vi "Test Control Packets.vi"() -> (0 "error out":errorcluster)   [LabVIEW 2013]
uses:
  <vilib>/addons/_JKI Toolkits/Caraya/classes/Test/Test.lvclass
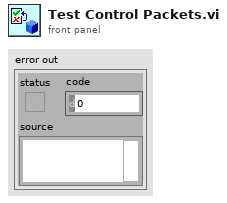
[diagram p1: front panel]
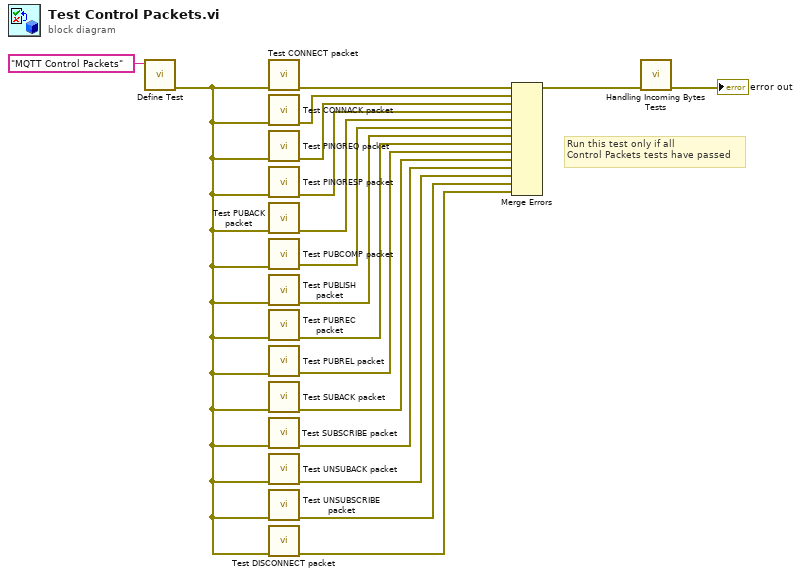
[diagram p0: block diagram]
diagram:
  # "Run this test only if all\nControl Packets tests have passed"
  n1 = call <vilib>:"Define Test.vi"("Label (VI Title)"="MQTT Control Packets") -> ("error out"=w1:errorcluster)  [unwired: 10 in]
  n2 = call "Test CONNECT packet.vi"("error in (no error)"=w1) -> ("error out"=w17:errorcluster)  [unwired: 10 in]
  n3 = call "Test CONNACK packet.vi"("error in (no error)"=w1) -> ("error out"=w16:errorcluster)  [unwired: 10 in]
  n4 = call "Test PINGREQ packet.vi"("error in (no error)"=w1) -> ("error out"=w15:errorcluster)  [unwired: 10 in]
  n5 = call "Test PINGRESP packet.vi"("error in (no error)"=w1) -> ("error out"=w14:errorcluster)  [unwired: 10 in]
  n6 = call "Test PUBACK packet.vi"("error in (no error)"=w1) -> ("error out"=w11:errorcluster)  [unwired: 10 in]
  n7 = call "Test PUBCOMP packet.vi"("error in (no error)"=w1) -> ("error out"=w10:errorcluster)  [unwired: 10 in]
  n8 = call "Test PUBLISH packet.vi"("error in (no error)"=w1) -> ("error out"=w9:errorcluster)  [unwired: 10 in]
  n9 = call "Test PUBREC packet.vi"("error in (no error)"=w1) -> ("error out"=w8:errorcluster)  [unwired: 10 in]
  n10 = call "Test PUBREL packet.vi"("error in (no error)"=w1) -> ("error out"=w7:errorcluster)  [unwired: 10 in]
  n11 = call "Test SUBACK packet.vi"("error in (no error)"=w1) -> ("error out"=w6:errorcluster)  [unwired: 10 in]
  n12 = call "Test SUBSCRIBE packet.vi"("error in (no error)"=w1) -> ("error out"=w2:errorcluster)  [unwired: 10 in]
  n13 = call "Test UNSUBACK packet.vi"("error in"=w1) -> ("error out"=w5:errorcluster)  [unwired: 10 in]
  n14 = call "Test UNSUBSCRIBE packet.vi"("error in"=w1) -> ("error out"=w4:errorcluster)  [unwired: 10 in]
  n15 = call "Test DISCONNECT packet.vi"("error in"=w1) -> ("error out"=w3:errorcluster)  [unwired: 10 in]
  n16 = Merge Errors(w17, w16, w15, w14, w11, w10, w9, w8, w7, w6, w2, w5, w4, w3) -> (w13:errorcluster)
  n17 = call "Handling Incoming Bytes Tests.vi"("error in (no error)"=w13) -> ("error out"=→"error out":errorcluster)  [unwired: 10 in]
